vi "AddMsg.vi"(1 "Result":bool=TRUE, 2 "添加消息":string, 3 "消息显示引用":refnum<vi>, 4 "消息Action":T1) -> (0 "消息":string)   [LabVIEW 2014]
uses:
  Controls/MsgAction.ctl
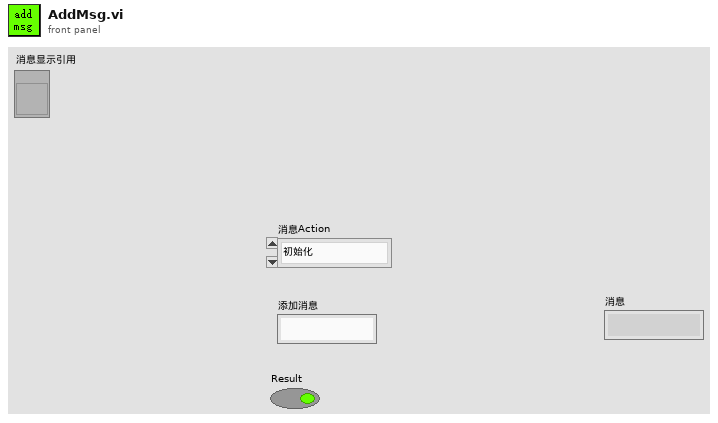
[diagram p1: front panel]
types:
  T1 = typedef "MsgAction.ctl" = enum16{"初始化", "添加消息", "区分结果添加消息", "清空消息", "获取消息"}
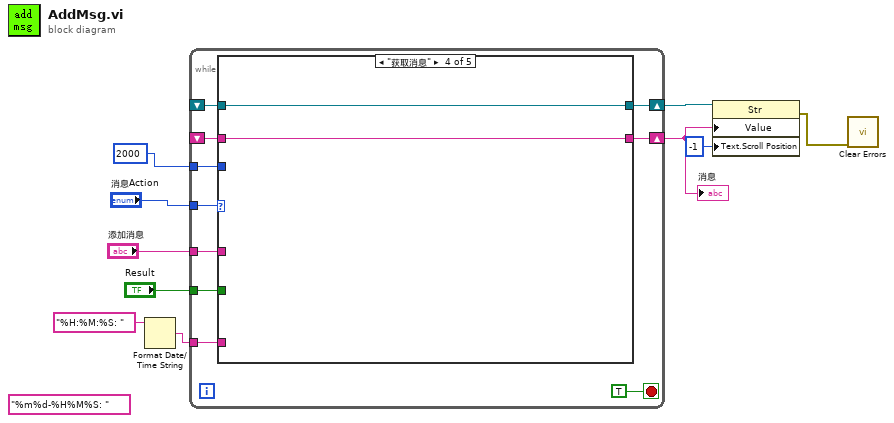
[diagram p0: block diagram]
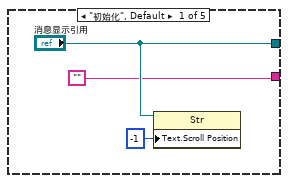
[diagram p2: hidden frame]
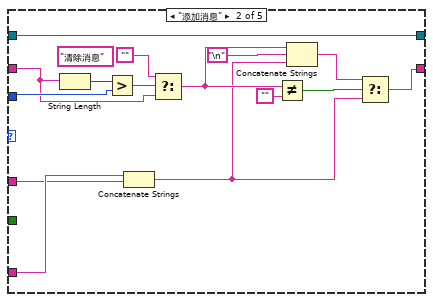
[diagram p3: hidden frame]
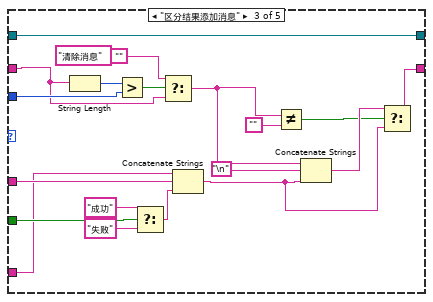
[diagram p4: hidden frame]
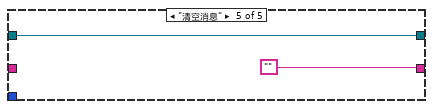
[diagram p5: hidden frame]
diagram:
  (unwired) "%m%d-%H%M%S: " ("time format string (%c)")
  n1 = Format Date/Time String(time format string (%c)="%H:%M:%S: ") -> (date/time string=w6:string)  [unwired: 2 in]
  n2 = while {
    tunnel: "消息Action" -> [w19]
    tunnel: "添加消息" -> [w17]
    shift-right: [w18] -> w2
    shift-left: _ -> [w16]
    tunnel: "Result" -> [w15]
    tunnel: w6 -> [w14]
    tunnel: 2000 -> [w13]
    shift-right: [w12] -> w4
    shift-left: _ -> [w11]
    stop <- TRUE stop-if-true
    n3 = case shown="\"获取消息\"" w19 {
      tunnel: ["" w34 w48 w59 ""] -> w18
      tunnel: w17 -> [_ w26 w50 _ _]
      tunnel: w16 -> [_ w30 w44 w59 _]
      tunnel: w15 -> [_ _ w51 _ _]
      tunnel: w14 -> [_ w27 w41 _ _]
      tunnel: w13 -> [_ w31 w46 _ _]
      tunnel: ["消息显示引用" w24 w39 w58 w60] -> w12
      tunnel: w11 -> [_ w24 w39 w58 w60]
      frame "初始化", Default {
        n4 = property class="Str"(reference="消息显示引用", "Text.Scroll Position"=-1 ("文本.滚动条位置")) -> ()  [unwired: 1 in, 2 out]
      }
      frame "添加消息" {
        (unwired) "清除消息" ("t")
        n5 = String Length(string=w30) -> (length=w33:i32)
        n6 = Greater?(x=w33, y=w31) -> (0:w32:bool)
        n7 = Concatenate Strings(w27, w26) -> (w25:string)
        n8 = Select(t="", s=w32, f=w30) -> (s? t:f=w29:string)
        n9 = Not Equal?(x=w29, y="") -> (x != y?=w35:bool)
        n10 = Concatenate Strings(w29, "\n", w25) -> (w36:string)
        n11 = Select(t=w36, s=w35, f=w25) -> (s? t:f=w34:string)
      }
      frame "区分结果添加消息" {
        (unwired) "清除消息" ("t")
        n12 = String Length(string=w44) -> (length=w47:i32)
        n13 = Greater?(x=w47, y=w46) -> (0:w45:bool)
        n14 = Select(t="成功", s=w51, f="失败") -> (s? t:f=w49:string)
        n15 = Select(t="", s=w45, f=w44) -> (s? t:f=w43:string)
        n16 = Concatenate Strings(w41, w50, w49) -> (w40:string)
        n17 = Not Equal?(x=w43, y="") -> (x != y?=w54:bool)
        n18 = Concatenate Strings(w43, "\n", w40) -> (w55:string)
        n19 = Select(t=w55, s=w54, f=w40) -> (s? t:f=w48:string)
      }
      frame "获取消息" {
      }
      frame "清空消息" {
      }
    }
  }
  "消息" <- w2
  n20 = property class="Str"(reference=w4, "Value"=w2, "Text.Scroll Position"=-1 ("文本.滚动条位置")) -> (error out=w1:errorcluster)  [unwired: 1 in, 1 out]
  n21 = call <vilib>:"Clear Errors.vi"("error in (no error)"=w1) -> ()  [unwired: 5 in, 2 out]
